vi "to_json.vi"(8 "error in":errorcluster, 11 "s3 in":refnum<class "s3.lvclass">) -> (0 "error out":errorcluster, 2 "json":string, 3 "s3 out":refnum<class "s3.lvclass">, 4 "Not Default":bool)   [LabVIEW 2020, in "datasources.lvlib" / "s3.lvclass"]
uses:
  s3.lvclass
  C:/code/labview-client/lv_src/Nominal Client/datasources/source/source.lvclass
  source/source.lvclass/source.ctl
  7d1f633d-aa90-401f-bff5-f9337493024e.vi
  b507f1fd-3569-41e4-9012-7a89e1841568.vi
  source/path.get.vi
  <vilib>/JDP Science/JSONtext/Variant to JSON Text.vi
  <vilib>/JDP Science/JSONtext/LVClass Serializer/JSONtext LVClass Serializer.lvclass
  s3.lvclass/s3.ctl
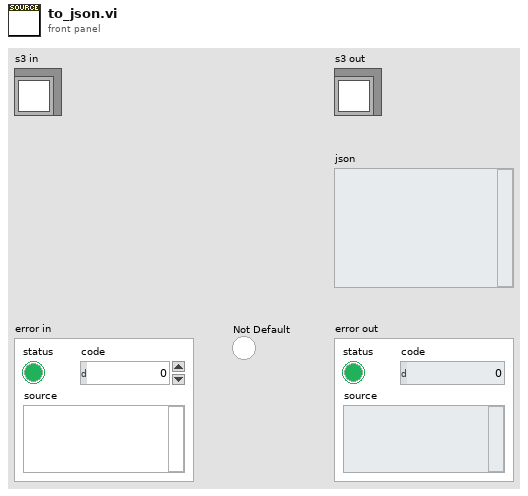
[diagram p1: front panel]
types:
  T1 = cluster{"type":string, "s3":cluster{"path":string}}
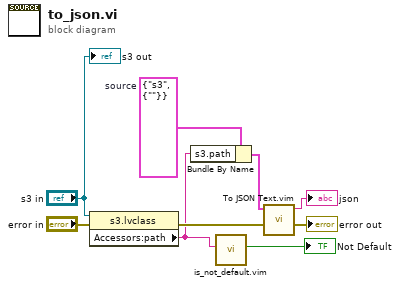
[diagram p0: block diagram]
diagram:
  w9 = T1 {"type"="s3", "s3"={"path"=""}}  # source
  n1 = property class="s3.lvclass"(reference="s3 in", error in="error in") -> (error out=w3:errorcluster, "Accessors:path"=w1:string)  [unwired: 1 out]
  n2 = Bundle By Name(cluster=w9, "s3.path"=w1) -> (w8:T1)
  n3 = call "is_not_default.vim"("data"=w1) -> ("Not Default"=→"Not Default":bool)  [unwired: 10 in]
  n4 = call "To JSON Text.vim"("error in (no error)"=w3, "Anything"=w8) -> ("error out"=→"error out":errorcluster, "<JSON>"=→"json":string)  [unwired: 8 in]
  "s3 out" <- "s3 in"
